vi "Arquitectura Basica de Control de Arduino.vi"() -> ()   [LabVIEW 2014]
uses:
  <vilib>/LabVIEW Interface for Arduino/Type Defs/Pin Mode.ctl
  <vilib>/LabVIEW Interface for Arduino/LabVIEW Interface for Arduino.lvlib
panel:
  in  "VISA resource name":refnum<visa-resource-name>
  out "Boolean 2":bool
  in  "Boolean":bool
  in  "stop":bool
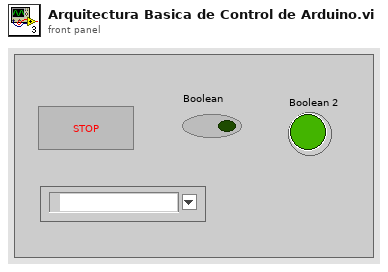
[diagram p1: front panel]
types:
  T1 = typedef "LabVIEW Interface for Arduino.lvlib/Pin Mode.ctl" = enum8{"Input", "Output"}
  T2 = typedef "LabVIEW Interface for Arduino.lvlib/Arduino Resource.ctl" = cluster{"VISA resource":refnum<visa-resource-name>, "Board Type":T3, "Connection Type":enum8{"USB / Serial"}, "Bytes Per Packet (15)":u8}
  T3 = typedef "LabVIEW Interface for Arduino.lvlib/Board Type.ctl" = enum16{"Uno", "Dimuelanove w/Atmega 328", "Mega 2560"}
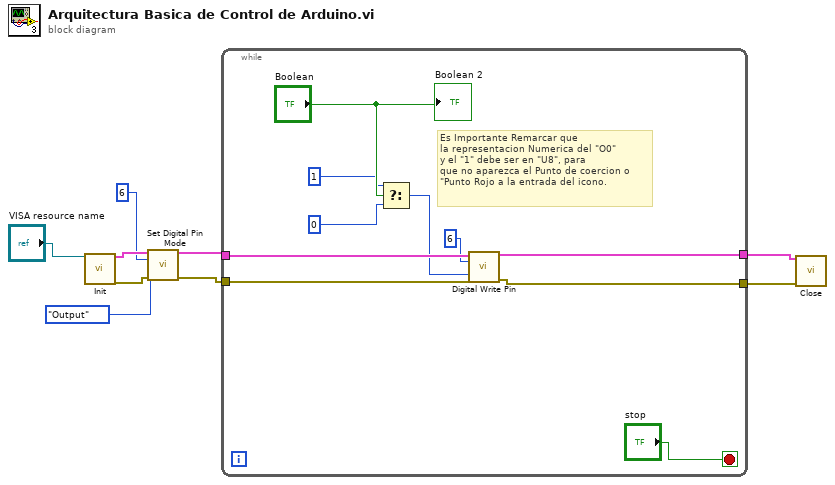
[diagram p0: block diagram]
diagram:
  n1 = call <vilib>:"Init.vi"("VISA resource"="VISA resource name") -> ("Arduino Resource"=w4:T2, "error out"=w3:errorcluster)  [unwired: 17 in]
  n2 = call <vilib>:"Set Digital Pin Mode.vi"("Arduino Resource"=w4, "Digital I/O Pin"=u8 6, "Pin Mode (Input)"=Pin_Mode."Output", "error in"=w3) -> ("Arduino Resource"=w5:T2, "error out"=w6:errorcluster)  [unwired: 10 in]
  n3 = while {
    tunnel: w5 -> [w19]
    tunnel: w6 -> [w18]
    tunnel: [w17] -> w9
    tunnel: [w16] -> w8
    stop <- "stop" stop-if-true
    # "Es Importante Remarcar que\nla representacion Numerica del \"O0\"\ny el \"1\" debe ser en \"U8\", para\nque no aparezca el Punto de coercion o \n\"Punto Rojo a la entrada del icono."
    n4 = Select(t=u8 1, s="Boolean", f=u8 0) -> (s? t:f=w14:u8)
    n5 = call <vilib>:"Digital Write Pin.vi"("Arduino Resource"=w19, "Digital I/O Pin (0)"=u8 6, "Value (0)"=w14, "error in"=w18) -> ("Arduino Resource"=w16:T2, "error out"=w17:errorcluster)  [unwired: 10 in]
    "Boolean 2" <- "Boolean"
  }
  n6 = call <vilib>:"Close.vi"("Arduino Resource"=w8, "error in"=w9) -> ()  [unwired: 13 in, 1 out]
